vi "CheckFrequency(SubVI).vi"(11 "wfm info":T1(array[cluster])) -> (3 "f (Hz)":dbl)   [LabVIEW 2020]
uses:
  <vilib>/Analysis/baseanly.llb/Mean (DBL).vi
  <vilib>/Analysis/NI_AALBase.lvlib
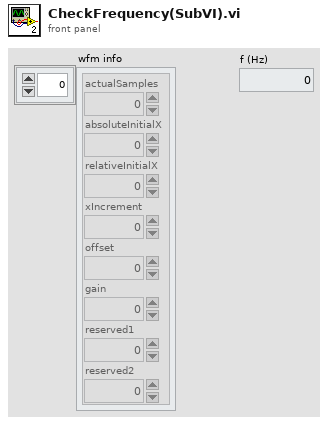
[diagram p1: front panel]
types:
  T1 = cluster{"actualSamples":i32, "absoluteInitialX":dbl, "relativeInitialX":dbl, "xIncrement":dbl, "offset":dbl, "gain":dbl, "reserved1":dbl, "reserved2":dbl}[]
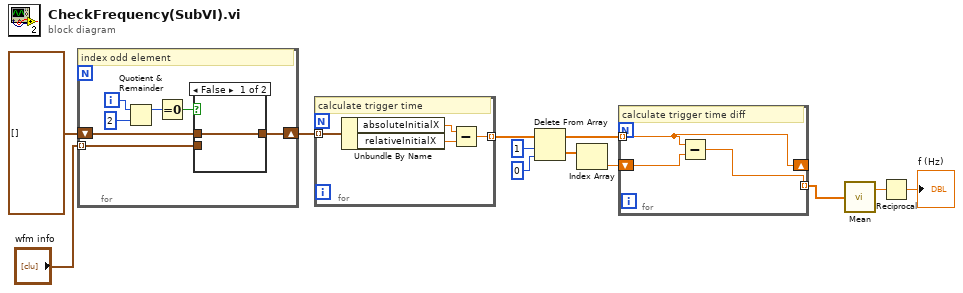
[diagram p0: block diagram]
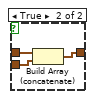
[diagram p2: hidden frame]
diagram:
  n1 = for {
    tunnel: "wfm info" -> [w15] mode=indexing
    shift-right: [w14] -> w8
    shift-left: T1 [] -> [w13]
    i -> [w19]
    # "index odd element"
    n2 = Quotient & Remainder(x=w19, y=2) -> (x-y*floor(x/y)=w17:i32)  [unwired: 1 out]
    n3 = Equal To 0?(x=w17) -> (x = 0?=w16:bool)
    n4 = case shown="False" w16 {
      tunnel: w15 -> [_ w23]
      tunnel: [w20 w22] -> w14
      tunnel: w13 -> [w20 w21]
      frame False {
      }
      frame True {
        n5 = Build Array (concatenate)(w21, w23) -> (w22:T1)
      }
    }
  }
  n6 = for {
    tunnel: w8 -> [w27] mode=indexing
    tunnel: [w24] -> w7 mode=indexing
    # "calculate trigger time"
    n7 = Unbundle By Name(w27) -> ("absoluteInitialX"=w26:dbl, "relativeInitialX"=w25:dbl)
    n8 = Subtract(x=w26, y=w25) -> (x-y=w24:dbl)
  }
  n9 = Delete From Array(array=w7, length=1, index=0) -> (deleted portion=w3:dbl[], array with subset deleted=w4:dbl[])
  n10 = Index Array(array=w3) -> (element=w2:dbl)  [unwired: 1 in]
  n11 = for {
    tunnel: w4 -> [w29] mode=indexing
    shift-right: [w29] -> _
    shift-left: w2 -> [w30]
    tunnel: [w28] -> w1 mode=indexing
    # "calculate trigger time diff"
    n12 = Subtract(x=w29, y=w30) -> (x-y=w28:dbl)
  }
  n13 = call-poly <vilib>:"Mean.vi"("X"=w1) -> ("mean"=w12:dbl)  [unwired: 1 out]
  n14 = Reciprocal(x=w12) -> (1/x=→"f (Hz)":dbl)
